vi "tc_array.vi"(0 "TC Label":string, 1 "output array 2":T1(array[cluster]), 2 "working":bool=TRUE, 5 "Temperature":dbl format="%#_13g", 7 "Graph ON/OFF":u32(colorbox)=6618880, 9 "Plot Color":u32(colorbox)=16860, 11 "Alarm String":string, 12 "index (row)":i32, 13 "index (col)":i32, 14 "AlarmColor":u32(colorbox)) -> (4 "output array":T1(array[cluster]))   [LabVIEW 2016]
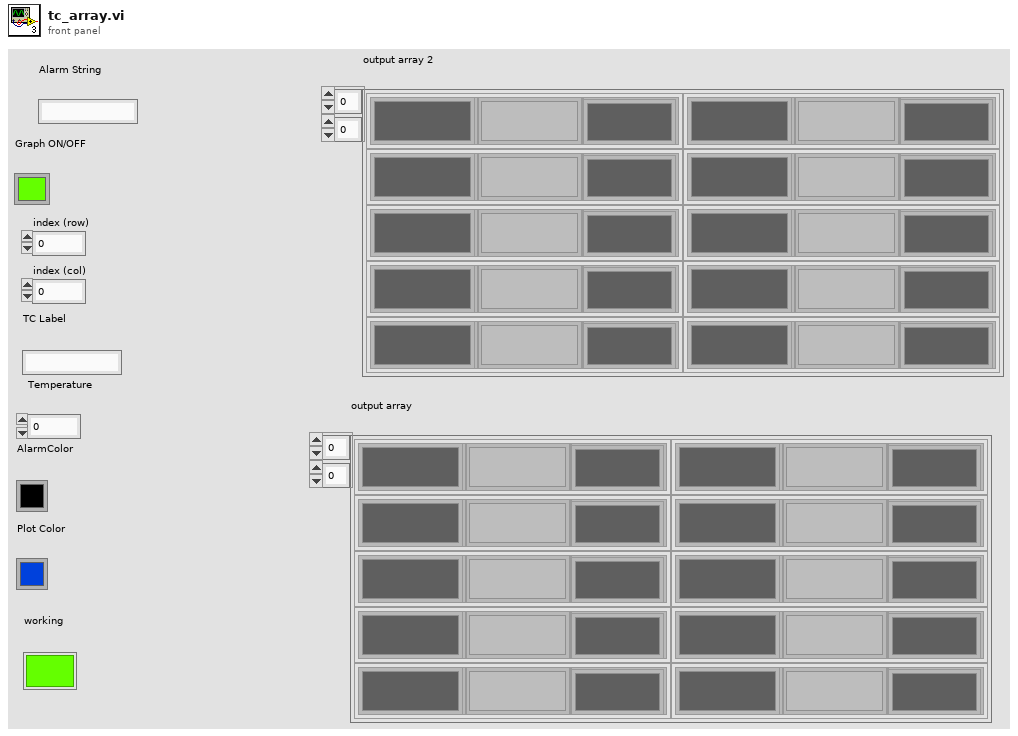
[diagram p1: front panel]
types:
  T1 = cluster{"TC Label":string, "Alarm Status":string, "Alarm Color":u32, "Temperature":string, "PlotColor":u32, "Graph On/Off":u32}[][]
  T2 = cluster{"TC Label":string, "Alarm Status":string, "Alarm Color":u32, "Temperature":string, "PlotColor":u32, "Graph On/Off":u32}
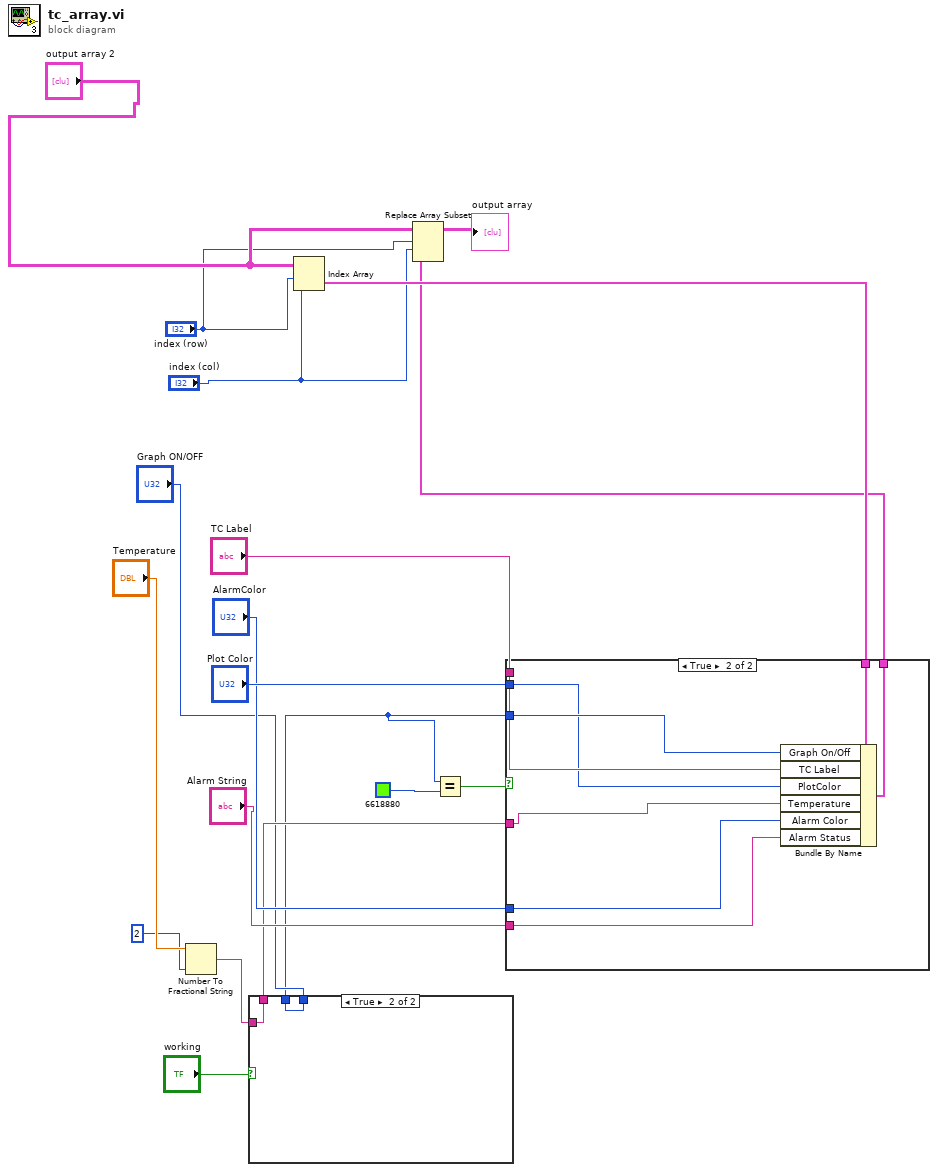
[diagram p0: block diagram]
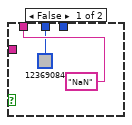
[diagram p2: hidden frame]
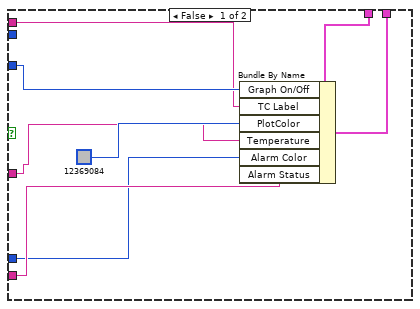
[diagram p3: hidden frame]
diagram:
  n1 = Number To Fractional String(number="Temperature", precision (6)=i16 2 ("width (-)")) -> (F-format string=w4:string)  [unwired: 2 in]
  n2 = case shown="True" "working" {
    tunnel: w4 -> [_ w23]
    tunnel: ["NaN" w23] -> w3
    tunnel: "Graph ON/OFF" -> [_ w22]
    tunnel: [u32 12369084 ("y") w22] -> w1
    frame False {
    }
    frame True {
    }
  }
  n3 = Index Array(array="output array 2", index (row)="index (row)", index (col)="index (col)") -> (element=w19:T2)
  n4 = Equal?(x=w1, y=u32 6618880) -> (x = y?=w11:bool)
  n5 = case shown="True" w11 {
    tunnel: w19 -> [w31 w39]
    tunnel: w1 -> [w29 w38]
    tunnel: "TC Label" -> [w27 w37]
    tunnel: "Plot Color" -> [_ w36]
    tunnel: "AlarmColor" -> [w25 w32]
    tunnel: "Alarm String" -> [w26 w35]
    tunnel: [w30 w34] -> w13
    tunnel: w3 -> [w24 w33]
    frame False {
      n6 = Bundle By Name(cluster=w31, "Graph On/Off"=w29, "TC Label"=w27, "PlotColor"=u32 12369084 ("Alarm Color"), "Temperature"=w24, "Alarm Color"=w25, "Alarm Status"=w26) -> (w30:T2)
    }
    frame True {
      n7 = Bundle By Name(cluster=w39, "Graph On/Off"=w38, "TC Label"=w37, "PlotColor"=w36, "Temperature"=w33, "Alarm Color"=w32, "Alarm Status"=w35) -> (w34:T2)
    }
  }
  n8 = Replace Array Subset(array="output array 2", new element=w13, index (row)="index (row)", index (col)="index (col)") -> (→"output array":T1)
